vi "FunctMgr.Load Return Data.vi"(6 "Ret Error":errorcluster, 8 "error in (no error)":errorcluster, 9 "Ret Data":variant, 10 "Ret ID":string, 11 "FunctMgr in":refnum<class "FunctMgr.lvclass">) -> (0 "error out":errorcluster, 1 "Found":bool, 3 "FunctMgr out":refnum<class "FunctMgr.lvclass">)   [LabVIEW 2018, in "FunctMgr.lvclass"]
uses:
  FunctMgr.lvclass
  <vilib>/KATE/SeqMgr/SeqMgr.Ret Msg Info.ctl
  <vilib>/KATE/Queues/Q.Msg Return Info.ctl
  <vilib>/KATE/Queues/Q.Element.ctl
  FunctMgr.lvclass/FunctMgr.ctl
  <vilib>/KATE/Queues/Queue Utils.lvlib
  <vilib>/KATE/SeqMgr/SeqMgr.lvlib
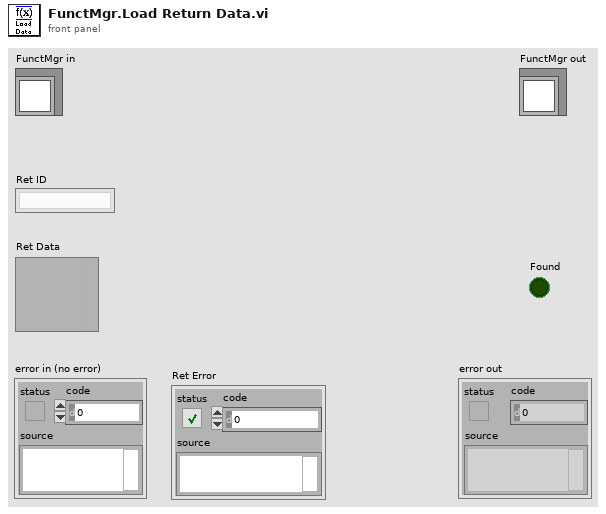
[diagram p1: front panel]
types:
  T1 = typedef "KATE_Lib.lvlib/SeqMgr.lvlib/SeqMgr.Ret Msg Info.ctl" = cluster{"ID":string, "Data":variant, "Ret Req":T2, "Error":errorcluster}
  T2 = typedef "KATE_Lib.lvlib/Queue Utils.lvlib/Q.Msg Return Info.ctl" = cluster{"Ret Q":refnum<queue>, "Ret Msg":T3, "SeqNum":i32}
  T3 = typedef "KATE_Lib.lvlib/Queue Utils.lvlib/Q.Element.ctl" = cluster{"Cmd":string, "Sub":string, "Data1":variant, "Data2":variant}
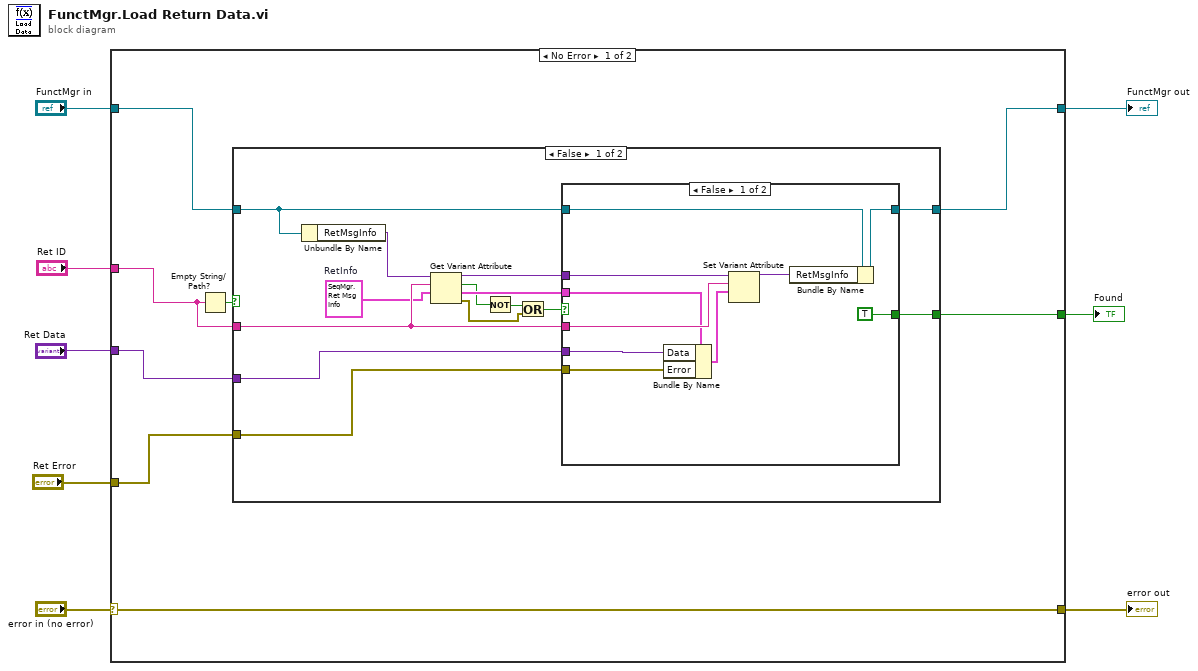
[diagram p0: block diagram]
diagram:
  n1 = case shown="No Error" "error in (no error)" {
    selector: "error in (no error)" -> [w9 w44]
    tunnel: [w9 w44] -> w7
    tunnel: [w11 w43] -> w5
    tunnel: "FunctMgr in" -> [w15 w43]
    tunnel: [w10 _] -> w4
    tunnel: "Ret Data" -> [w13 _]
    tunnel: "Ret ID" -> [w14 _]
    tunnel: "Ret Error" -> [w12 _]
    frame No Error {
      n2 = Empty String/Path?(string/path=w14) -> (empty?=w16:bool)
      n3 = case shown="False" w16 {
        tunnel: [w30 w42] -> w11
        tunnel: w15 -> [w29 w42]
        tunnel: w14 -> [w26 _]
        tunnel: w13 -> [w23 _]
        tunnel: [w18 _] -> w10
        tunnel: w12 -> [w17 _]
        frame False {
          w24 = T1 {"ID"="", "Data"=variant, "Ret Req"={"Ret Q"=refnum, "Ret Msg"={"Cmd"="", "Sub"="", "Data1"=variant, "Data2"=variant}, "SeqNum"=0}, "Error"={"status"=FALSE, "code"=0, "source"=""}}  # RetInfo
          n4 = Unbundle By Name(w29) -> ("RetMsgInfo"=w28:variant)
          n5 = Get Variant Attribute(Variant=w28, name=w26, default value (empty Variant)=w24) -> (duplicate Variant=w27:variant, found=w22:bool, value=w25:T1, error out=w20:errorcluster)  [unwired: 1 in]
          n6 = Not(x=w22) -> (.not. x?=w21:bool)
          n7 = Or(x=w21, y=w20) -> (x .or. y?=w19:bool)
          n8 = case shown="False" w19 {
            tunnel: [w40 w41] -> w30
            tunnel: w29 -> [w39 w41]
            tunnel: w27 -> [w38 _]
            tunnel: w26 -> [w37 _]
            tunnel: w25 -> [w36 _]
            tunnel: w23 -> [w35 _]
            tunnel: [TRUE _] -> w18
            tunnel: w17 -> [w31 _]
            frame False {
              n9 = Bundle By Name(cluster=w36, "Data"=w35, "Error"=w31) -> (w34:T1)
              n10 = Set Variant Attribute(Variant=w38, name=w37, value=w34) -> (Variant out=w33:variant)  [unwired: 1 in, 2 out]
              n11 = Bundle By Name(cluster=w39, "RetMsgInfo"=w33) -> (w40:refnum<class "FunctMgr.lvclass">)
            }
            frame True {
              # "Do nothing\nError or not found"
            }
          }
        }
        frame True {
          # "Do nothing\nEmpty ID"
        }
      }
    }
    frame Error {
    }
  }
  "error out" <- w7
  "FunctMgr out" <- w5
  "Found" <- w4
